vi "Get Plugin Location.vi"() -> (3 "Plugin Directory":path)   [LabVIEW 2021, in "CIFPluginManager.lvclass"]
uses:
  CIFPluginManager.lvclass
  CIFPluginManager.lvclass/CIFPluginManager.ctl
  CIFUtilities/CIFConfigurationFile/CIF Configuration File.lvlib
  CIFUtilities/CIFConfigurationFile/typedef/Location Type.ctl
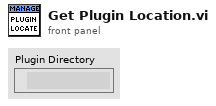
[diagram p1: front panel]
types:
  T1 = typedef "CIF Configuration File.lvlib/Location Type.ctl" = enum16{"Config File", "Manager", "Protos", "Plugins", "UI Plugins", "Logs"}
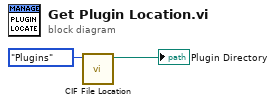
[diagram p0: block diagram]
diagram:
  n1 = call "CIF File Location.vi"("LocationType"=Location_Type."Plugins") -> ("Location"=→"Plugin Directory":path)  [unwired: 10 in]
